vi "Bool_Pulse on off.vi"(5 "Pulse time(S) In":dbl=2.0 format="%.2g", 6 "Pulse on input Rise(t) Fall(f) In":bool=TRUE, 7 "Hi(t) Lo(f) Pulse In":bool=TRUE, 8 "Enable timmer In":bool=TRUE, 9 "input In":bool) -> (0 "input Fall Out":bool, 1 "input Rise Out":bool, 2 "Output Out":bool, 3 "Pulse Output Out":bool, 4 "Time left (S) Out":dbl)   [LabVIEW 2015]
panel:
  in  "stop":bool=TRUE
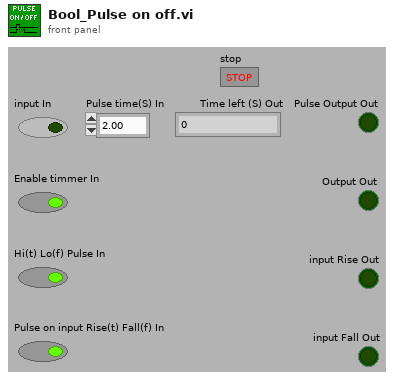
[diagram p1: front panel]
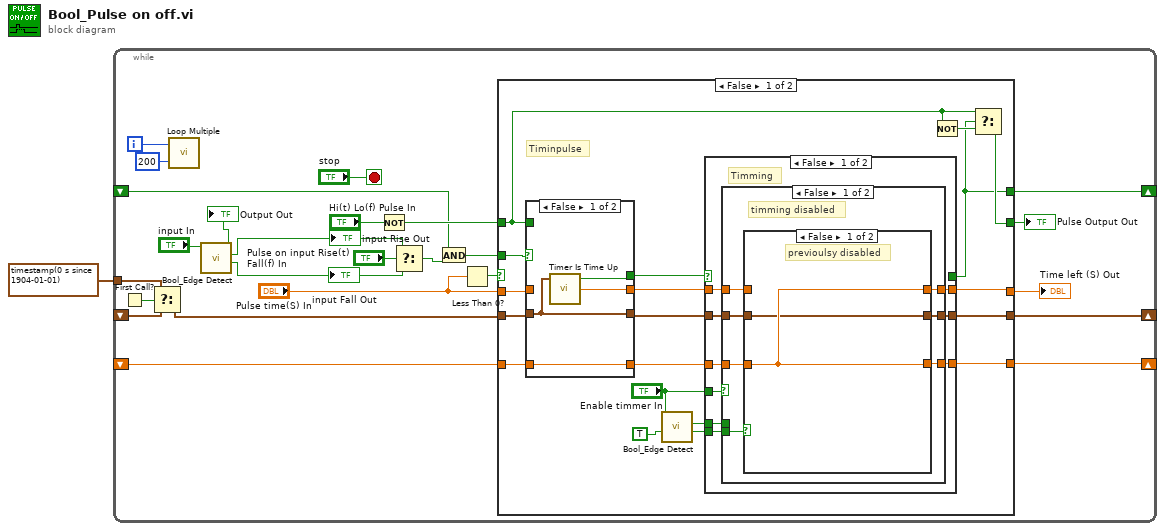
[diagram p0: block diagram]
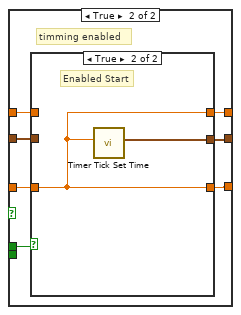
[diagram p3: hidden frame]
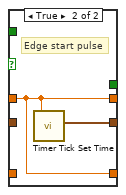
[diagram p6: hidden frame]
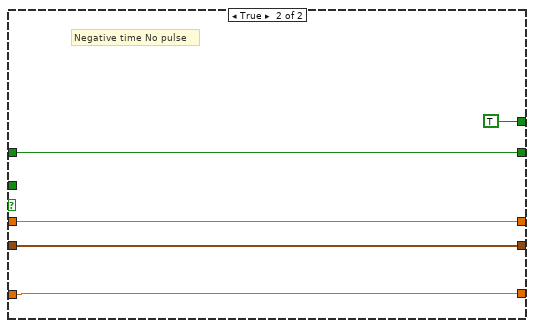
[diagram p7: hidden frame]
diagram:
  n1 = while {
    shift-right: [w17] -> _
    shift-left: _ -> [w16]
    tunnel: timestamp(0 s since 1904-01-01) ("t") -> [w11]
    shift-right: [w8] -> _
    shift-left: _ -> [w6]
    shift-right: [w3] -> _
    shift-left: _ -> [w2]
    i -> [w10]
    stop <- "stop" stop-if-true
    n2 = First Call?() -> (First Call?: T/F=w23:bool)
    n3 = Select(t=w11, s=w23, f=w16) -> (s? t:f=w18:timestamp)
    n4 = call "Loop Multiple.vi"("millisecond multiple"=u32 200, "Iteration"=w10) -> ()  [unwired: 1 in]
    n5 = call "Bool_Edge Detect.vi"("Input/Set"="input In") -> ("Fall"=w13:bool, "Rise"=w14:bool, "Output"=→"Output Out":bool)  [unwired: 7 in, 1 out]
    "input Fall Out" <- w13
    "input Rise Out" <- w14
    n6 = Not(x="Hi(t) Lo(f) Pulse In") -> (.not. x?=w21:bool)
    n7 = Select(t=w14, s="Pulse on input Rise(t) Fall(f) In", f=w13) -> (s? t:f=w12:bool)
    n8 = And(x=w6, y=w12) -> (x .and. y?=w7:bool)
    n9 = Less Than 0?(x="Pulse time(S) In") -> (x < 0?=w4:bool)
    n10 = case shown="False" w4 {
      tunnel: w21 -> [w41 w90]
      tunnel: [w40 w90] -> w20
      tunnel: [w37 w91] -> w19
      tunnel: w18 -> [w45 w92]
      tunnel: [w36 w92] -> w17
      tunnel: "Pulse time(S) In" -> [w44 w91]
      tunnel: [w39 TRUE ("Time Complete")] -> w8
      tunnel: w7 -> [w43 _]
      tunnel: [w29 w88] -> w3
      tunnel: w2 -> [w27 w88]
      frame False {
        # "Timinpulse"
        n11 = case shown="False" w43 {
          tunnel: w41 -> [_ _]
          tunnel: [w85 w86] -> w38
          tunnel: w45 -> [w84 _]
          tunnel: [w84 w87] -> w35
          tunnel: w44 -> [_ w86]
          tunnel: [w83 _] -> w33
          tunnel: [w82 w86] -> w28
          tunnel: w27 -> [w82 _]
          frame False {
            n12 = call "Timer Is Time Up.vi"("Finish Time"=w84) -> ("Time left (S)"=w85:dbl, "Time Complete"=w83:bool)  [unwired: 2 in, 1 out]
          }
          frame True {
            # "Edge start pulse"
            n13 = call "Timer Tick Set Time.vi"("Seconds till stop (S)"=w86) -> ("Finish Time"=w87:timestamp)  [unwired: 5 in, 1 out]
          }
        }
        n14 = call "Bool_Edge Detect.vi"("Initial State"=TRUE, "Input/Set"="Enable timmer In") -> ("Fall"=w32:bool, "Rise"=w30:bool)  [unwired: 6 in, 2 out]
        n15 = case shown="False" w33 {
          selector: w33 -> [_ w81]
          tunnel: [_ w81] -> w39
          tunnel: [w47 w80] -> w37
          tunnel: w38 -> [w51 w80]
          tunnel: w35 -> [w53 w79]
          tunnel: [w52 w79] -> w36
          tunnel: w32 -> [w50 _]
          tunnel: "Enable timmer In" -> [w54 _]
          tunnel: w30 -> [w49 _]
          tunnel: [w48 w78] -> w29
          tunnel: w28 -> [w46 w78]
          frame False {
            # "Timming"
            n16 = case shown="False" w54 {
              tunnel: w53 -> [w60 w67]
              tunnel: [w56 w71] -> w52
              tunnel: w51 -> [w59 w69]
              tunnel: w50 -> [w61 _]
              tunnel: w49 -> [_ w72]
              tunnel: [w58 w66] -> w48
              tunnel: [w57 w68] -> w47
              tunnel: w46 -> [w55 w70]
              frame False {
                # "timming disabled"
                n17 = case shown="False" w61 {
                  tunnel: w60 -> [w62 w64]
                  tunnel: w59 -> [_ w65]
                  tunnel: [w63 w65] -> w58
                  tunnel: [w63 w65] -> w57
                  tunnel: [w62 w64] -> w56
                  tunnel: w55 -> [w63 _]
                  frame False {
                    # "previoulsy disabled"
                  }
                  frame True {
                    # "Disabled start"
                  }
                }
              }
              frame True {
                # "timming enabled"
                n18 = case shown="True" w72 {
                  tunnel: [w74 w77] -> w71
                  tunnel: w70 -> [w73 w76]
                  tunnel: w69 -> [w75 _]
                  tunnel: [w75 w76] -> w68
                  tunnel: w67 -> [w74 _]
                  tunnel: [w73 w76] -> w66
                  frame False {
                    # "Previously enabled"
                  }
                  frame True {
                    # "Enabled Start"
                    n19 = call "Timer Tick Set Time.vi"("Seconds till stop (S)"=w76) -> ("Finish Time"=w77:timestamp)  [unwired: 5 in, 1 out]
                  }
                }
              }
            }
          }
          frame True {
            # "not timming"
          }
        }
        n20 = Not(x=w41) -> (.not. x?=w42:bool)
        n21 = Select(t=w41, s=w39, f=w42) -> (s? t:f=w40:bool)
      }
      frame True {
        # "Negative time No pulse"
      }
    }
    "Pulse Output Out" <- w20
    "Time left (S) Out" <- w19
  }
